vi "Report.vi"() -> ()   [LabVIEW 2017]
uses:
  <vilib>/Utility/miscctls.llb/LVRowAndColumnUnsignedTypeDef.ctl
  <vilib>/addons/database/Connection.llb/DB Tools Open Connec (String).vi
  <vilib>/Utility/file.llb/Write Delimited Spreadsheet (string).vi
  Global/Global 1.vi
  <vilib>/addons/database/NI_Database_API.lvlib
  <vilib>/Utility/NIReport.llb/NI_report.lvclass
  <vilib>/Utility/NIReport.llb/Append Text Table to Report (wrap).vi
panel:
  out "reposr save header":string[](array[string])
  in  "SELECT REPORT TYPE":string(combo)="WITHOUT TRECIABILITY"
  out "error out":errorcluster
  in  "error in (no error)":errorcluster
  in  "GET REPORT":bool
  in  "EXIT":bool
  in  "EXPORT TO EXCEL":bool
  in  "TO":timestamp format="%<%x>T"
  in  "FROM":timestamp format="%<%x>T"
  in  "BARCODE":string
  in  "TYPE":string(combo)="DATE TIME"
  in  "STATION WISE":string(combo)="OP 10"
  out "Table":string[][](table)
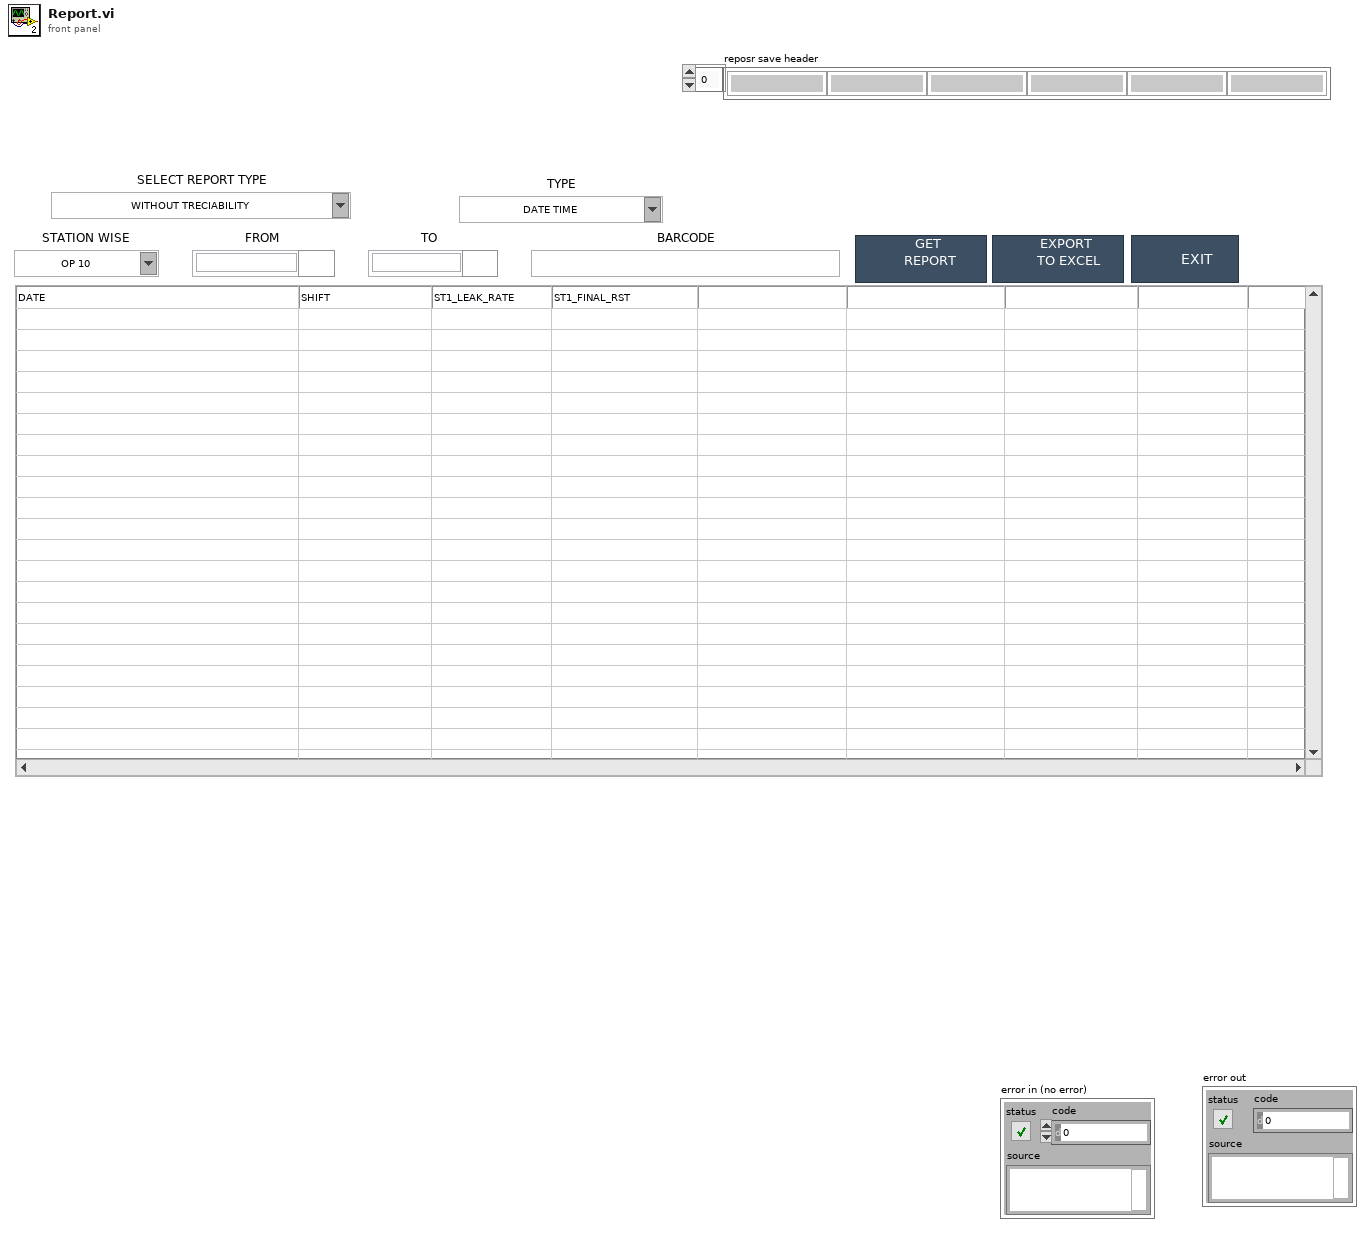
[diagram p1: front panel]
types:
  T1 = typedef "NI_Database_API.lvlib/Conn ObjectReference.ctl" = refnum<k1>
  T2 = typedef "LVRowAndColumnUnsignedTypeDef.ctl" = cluster{"Row":u32, "Column":u32}
  T3 = enum16{"Standard Report", "HTML", "Word", "Excel"}
  T4 = enum16{"maximized", "minimized", "normal", "no change"}
  T5 = enum32{"invalid app kind", "Development System", "Run Time System", "Student Edition", "Embedded LabVIEW", "Evaluation", "Custom"}
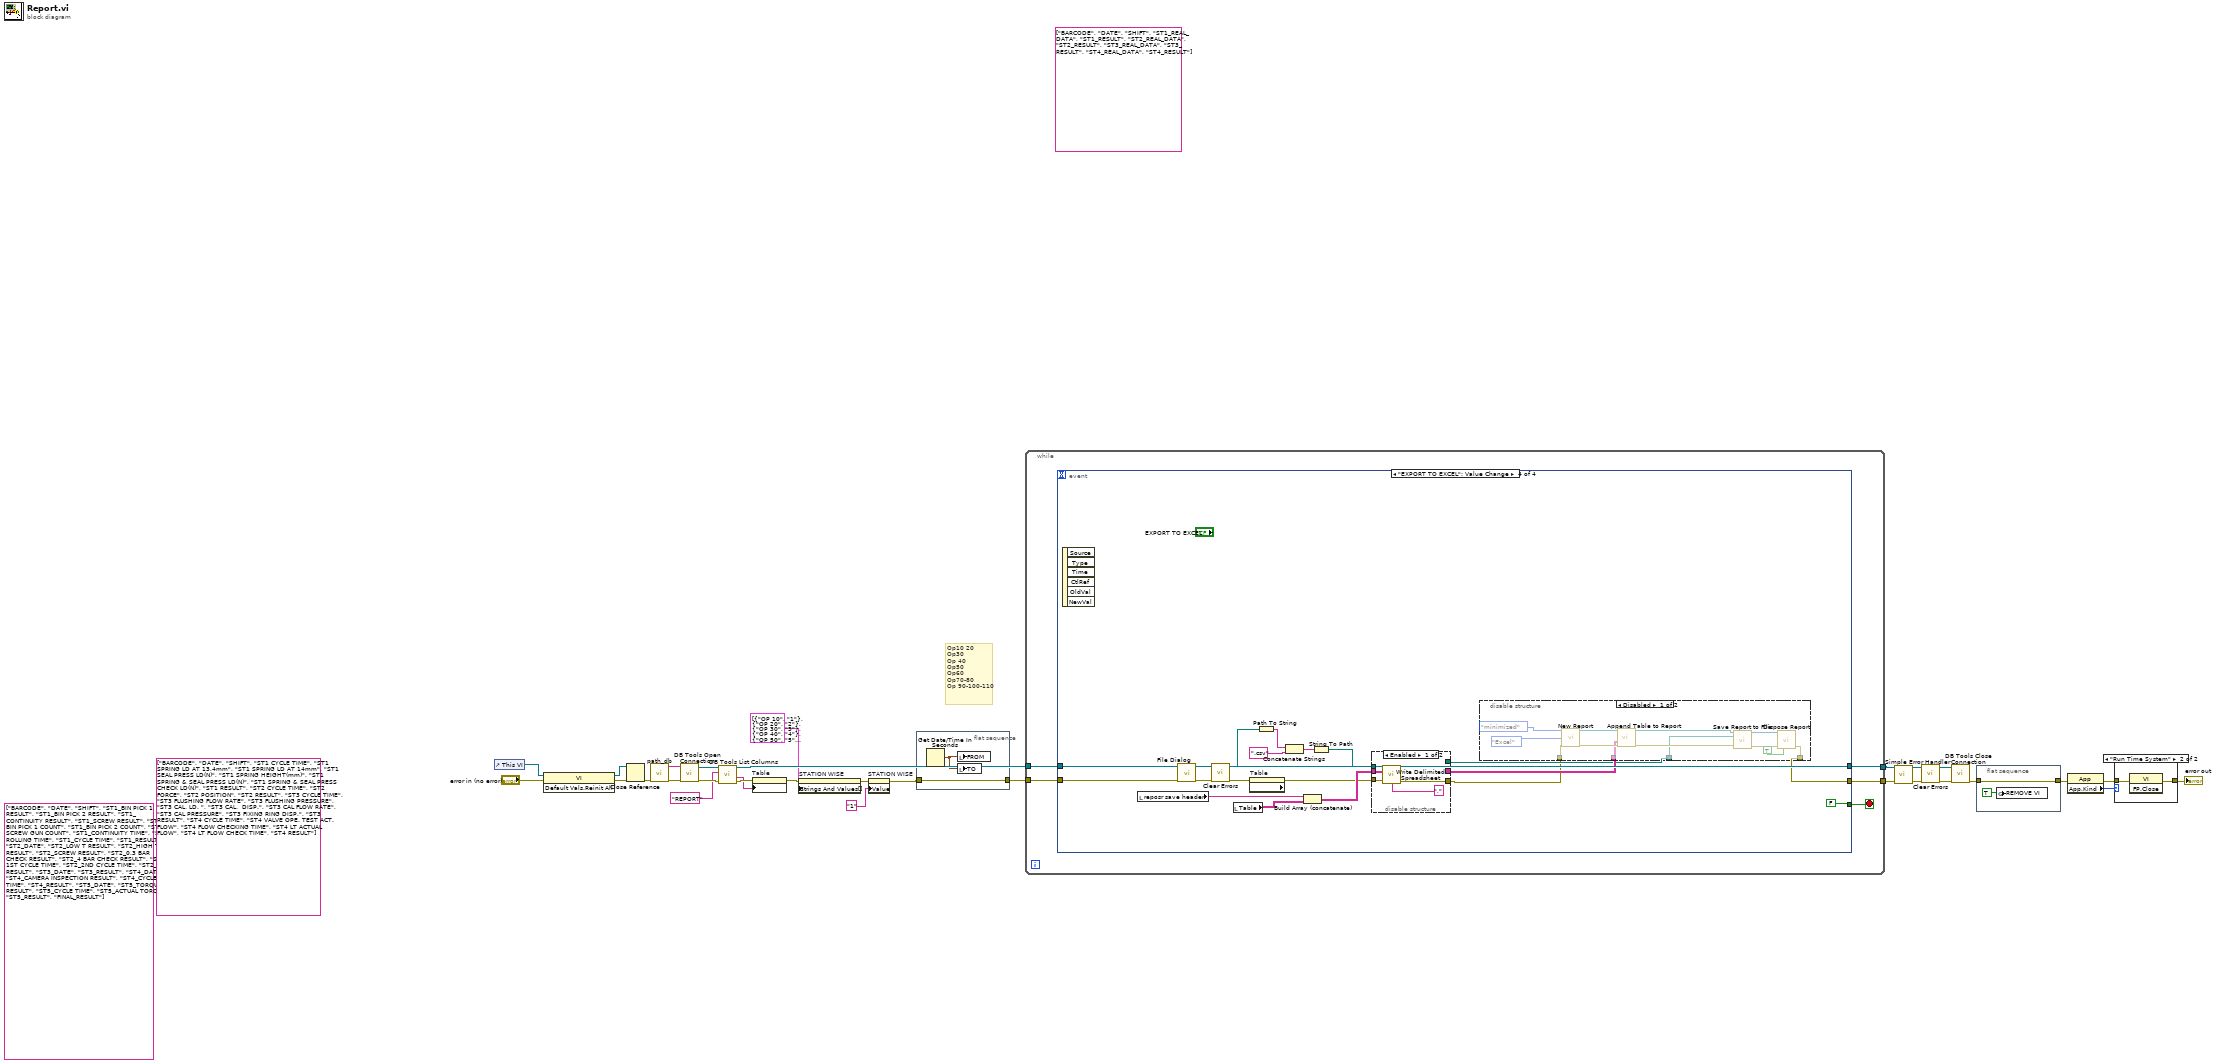
[diagram p0: block diagram]
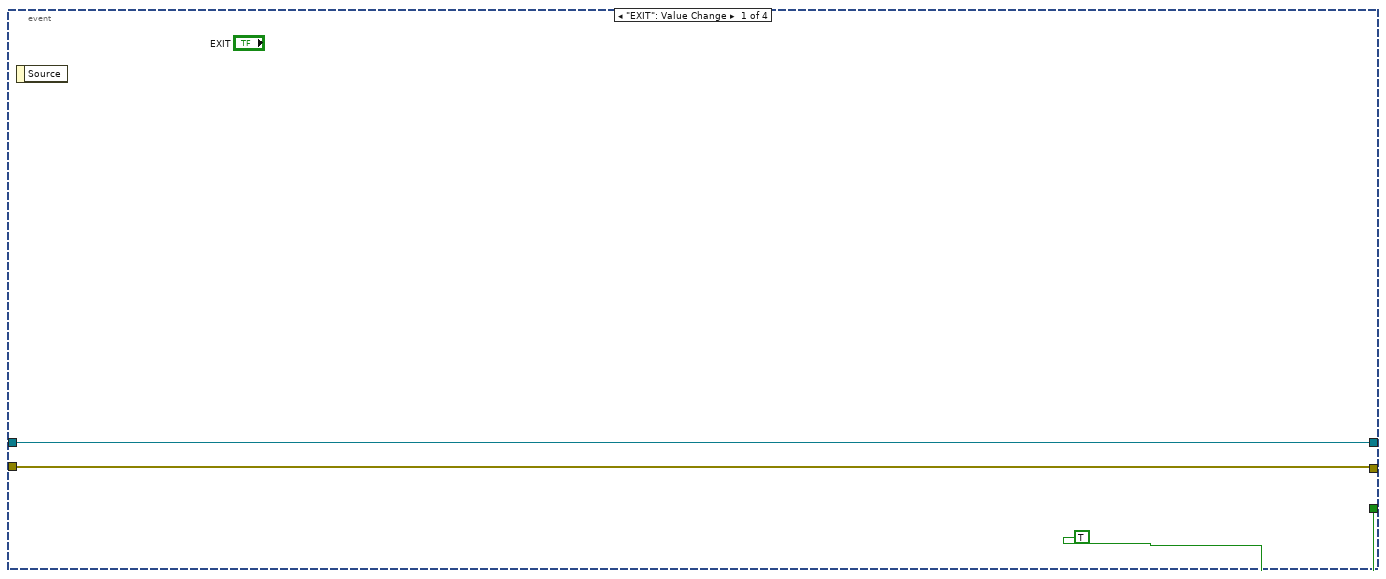
[diagram p2: hidden frame]
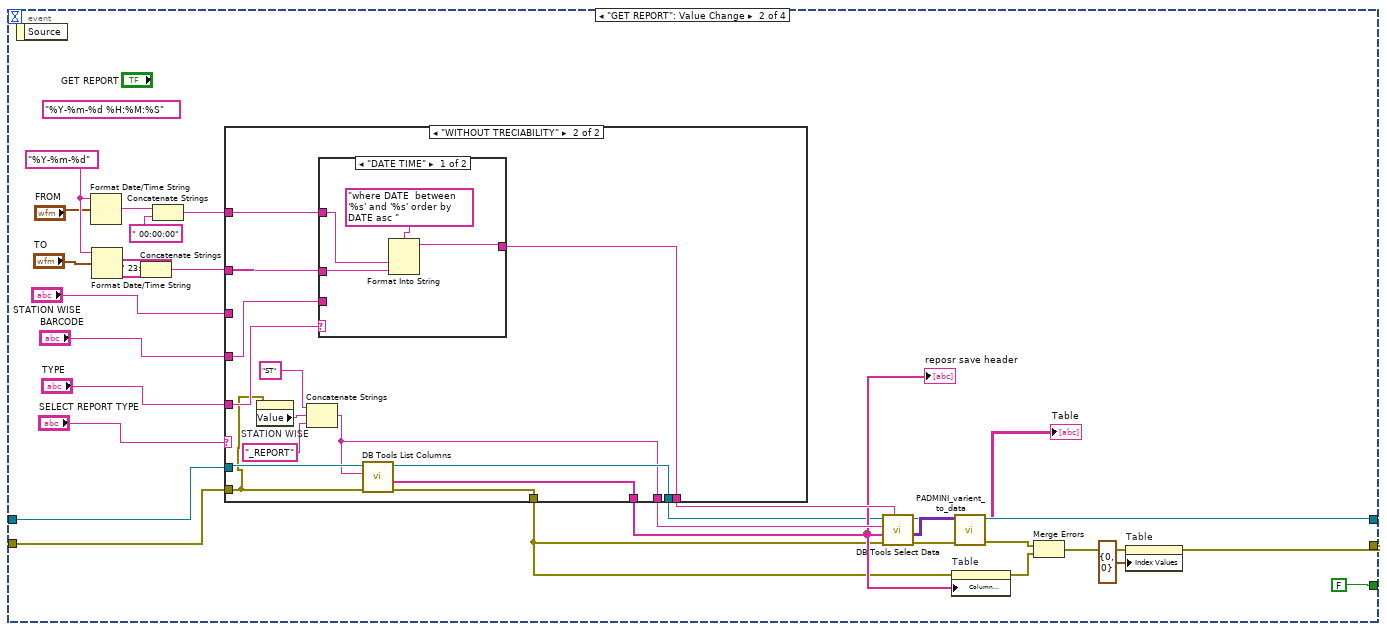
[diagram p3: hidden frame]
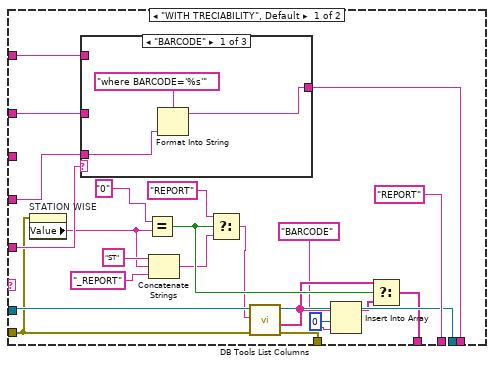
[diagram p4: hidden frame]
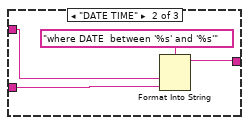
[diagram p5: hidden frame]
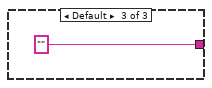
[diagram p6: hidden frame]
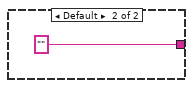
[diagram p7: hidden frame]
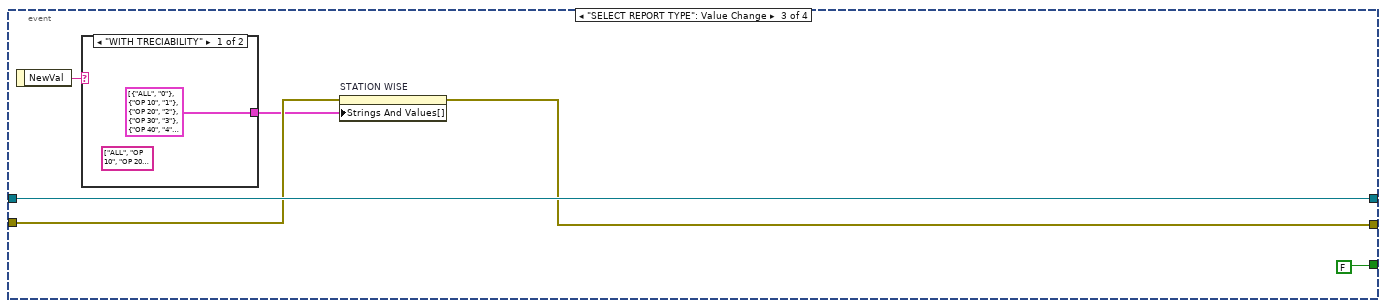
[diagram p8: hidden frame]
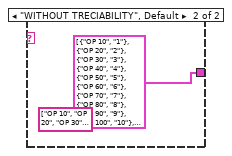
[diagram p9: hidden frame]
diagram:
  (unwired) string[] ["BARCODE", "DATE", "SHIFT", "ST1_REAL_DATA", "ST1_RESULT", "ST2_REAL_DATA", "ST2_RESULT", "ST3_REAL_DATA", "ST3_RESULT", "ST4_REAL_DATA", "ST4_RESULT"]
  (unwired) string[] ["BARCODE", "DATE", "SHIFT", "ST1_BIN PICK 1 RESULT", "ST1_BIN PICK 2 RESULT", "ST1_CONTINUITY RESULT", "ST1_SCREW RESULT", "ST1_BIN PICK 1 COUNT", "ST1_BIN PICK 2 COUNT", "ST1_SCREW GUN COUNT", "ST1_CONTINUITY TIME", "ST1_ROLLING TIME", "ST1_CYCLE TIME", "ST1_RESULT", "ST2_DATE", "ST2_LOW T RESULT", "ST2_HIGH T RESULT", "ST2_SCREW RESULT", "ST2_0.3 BAR CHECK RESULT", "ST2_4 BAR CHECK RESULT", "ST2_1ST CYCLE TIME", "ST2_2ND CYCLE TIME", "ST2_RESULT", "ST3_DATE", "ST3_RESULT", "ST4_DATE", "ST4_CAMERA INSPECTION RESULT", "ST4_CYCLE TIME", "ST4_RESULT", "ST5_DATE", "ST5_TORQUE RESULT", "ST5_CYCLE TIME", "ST5_ACTUAL TORQUE", "ST5_RESULT", "FINAL_RESULT"]
  (unwired) string[] ["BARCODE", "DATE", "SHIFT", "ST1 CYCLE TIME", "ST1 SPRING LD AT 13.4mm", "ST1 SPRING LD AT 14mm", "ST1 SEAL PRESS LD(N)", "ST1 SPRING HEIGHT(mm)", "ST1 SPRING & SEAL PRESS LD(N)", "ST1 SPRING & SEAL PRESS CHECK LD(N)", "ST1 RESULT", "ST2 CYCLE TIME", "ST2 FORCE", "ST2 POSITION", "ST2 RESULT", "ST3 CYCLE TIME", "ST3 FLUSHING FLOW RATE", "ST3 FLUSHING PRESSURE", "ST3 CAL. LD. ", "ST3 CAL.  DISP.", "ST3 CAL FLOW RATE", "ST3 CAL PRESSURE", "ST3 FIXING RING DISP.", "ST3 RESULT", "ST4 CYCLE TIME", "ST4 VALVE OPE. TEST ACT. FLOW", "ST4 FLOW CHECKING TIME", "ST4 LT ACTUAL FLOW", "ST4 LT FLOW CHECK TIME", "ST4 RESULT"]
  # "Op10 20\nOp30\nOp 40\nOp50\nOp60\nOp70-80\nOp 90-100-110"
  n1 = control-ref of="This VI"() -> (w28:refnum<vi>)
  n2 = invoke class="VI" method="Default Vals.Reinit All"(reference=w28, error in="error in (no error)") -> (reference out=w26:refnum<vi>, error out=w25:errorcluster)  [unwired: 1 in, 1 out]
  n3 = Close Reference(reference=w26, error in (no error)=w25) -> (error out=w15:errorcluster)
  n4 = call "path_db.vi"("error in"=w15) -> ("error out"=w17:errorcluster, "resulting string"=w16:string)  [unwired: 9 in]
  n5 = call-poly <vilib>:"DB Tools Open Connection.vi"("error in (no error)"=w17, "connection information"=w16) -> ("error out"=w10:errorcluster, "connection reference"=w7:T1)  [unwired: 6 in]
  n6 = call <vilib>:"DB Tools List Columns.vi"("error in (no error)"=w10, "table"="REPORT", "connection reference"=w7) -> ("error out"=w9:errorcluster, "columns"=w6:string[], "connection reference out"=w8:T1)  [unwired: 1 in, 1 out]
  n7 = property on="Table" class="Tbl (strict)"(error in=w9, "Column Headers[]"=w6) -> (error out=w12:errorcluster)  [unwired: 1 in, 1 out]
  n8 = property on="STATION WISE" class="CmbBox"(error in=w12, "Strings And Values[]"=cluster{"String":string, "Value":string}[] [{"String"="OP 10", "Value"="1"}, {"String"="OP 20", "Value"="2"}, {"String"="OP 30", "Value"="3"}, {"String"="OP 40", "Value"="4"}, {"String"="OP 50", "Value"="5"}, {"String"="OP 60", "Value"="6"}, {"String"="OP 70", "Value"="7"}, {"String"="OP 80", "Value"="8"}, {"String"="OP 90", "Value"="9"}, {"String"="OP 100", "Value"="10"}, {"String"="OP 110", "Value"="11"}] ("Strings And Values [] 2")) -> (error out=w3:errorcluster)  [unwired: 1 in, 1 out]
  n9 = property on="STATION WISE" class="CmbBox"(error in=w3, "Value"="1") -> (error out=w2:errorcluster)  [unwired: 1 in, 1 out]
  n10 = flat-sequence {
    tunnel: w2 -> [w29]
    tunnel: [w29] -> w11
    frame #0 {
      n11 = Get Date/Time In Seconds() -> (seconds since 1Jan1904=w30:timestamp)
      n12 = local write "FROM"(w30) -> ()
      n13 = local write "TO"(w30) -> ()
    }
  }
  n14 = while {
    tunnel: [w32] -> w18
    tunnel: w11 -> [w34]
    tunnel: w8 -> [w33]
    tunnel: [w31] -> w13
    stop <- w35 stop-if-true
    n15 = event shown="[3] \"EXPORT TO EXCEL\": Value Change" {
      selector: _ -> [_ _ _ _]
      dyn-events: _ -> [_ _ _ _]
      timeout: _ -> [_ _ _ _]
      tunnel: [TRUE FALSE FALSE FALSE] -> w35
      tunnel: w34 -> [w36 w45 w122 w132]
      tunnel: w33 -> [w37 w43 w124 w143]
      tunnel: [w37 w51 w124 w143] -> w31
      tunnel: [w36 w52 w119 w129] -> w32
      event "EXIT": Value Change {
        n16 = event-data() -> ()  [unwired: 1 in, 1 out]
      }
      event "GET REPORT": Value Change {
        (unwired) "%Y-%m-%d %H:%M:%S" ("time format string (%c)")
        w65 = "%Y-%m-%d" ("time format string (%c)")
        n17 = event-data() -> ()  [unwired: 1 in, 1 out]
        n18 = Format Date/Time String(time format string (%c)=w65, seconds (now)="FROM") -> (date/time string=w59:string)  [unwired: 1 in]
        n19 = Format Date/Time String(time format string (%c)=w65, seconds (now)="TO") -> (date/time string=w56:string)  [unwired: 1 in]
        n20 = Concatenate Strings(w56, " 23:59:59" ("time format string (%c)")) -> (w55:string)
        n21 = Concatenate Strings(w59, " 00:00:00" ("time format string (%c)")) -> (w58:string)
        n22 = case shown="\"WITHOUT TRECIABILITY\"" "SELECT REPORT TYPE" {
          tunnel: "TYPE" -> [w91 w113]
          tunnel: [w90 w112] -> w67
          tunnel: "BARCODE" -> [w89 w111]
          tunnel: w58 -> [w88 w110]
          tunnel: w55 -> [w87 w106]
          tunnel: "STATION WISE" -> [_ _]
          tunnel: ["REPORT" w101] -> w46
          tunnel: w45 -> [w69 w100]
          tunnel: [w83 w105] -> w39
          tunnel: [w79 w104] -> w44
          tunnel: w43 -> [w85 w103]
          tunnel: [w84 w102] -> w42
          frame "WITH TRECIABILITY", Default {
            n23 = property on="STATION WISE" class="CmbBox"(error in=w69) -> ("Value"=w70:string)  [unwired: 1 in, 2 out]
            n24 = case shown="\"BARCODE\"" w91 {
              tunnel: [w93 w97 ""] -> w90
              tunnel: w89 -> [w92 _ _]
              tunnel: w88 -> [_ w96 _]
              tunnel: w87 -> [_ w95 _]
              frame "BARCODE" {
                n25 = Format Into String(format string="where BARCODE='%s'", w92) -> (resulting string=w93:string)  [unwired: 2 in, 1 out]
              }
              frame "DATE TIME" {
                n26 = Format Into String(format string="where DATE  between '%s' and '%s'", w96, w95) -> (resulting string=w97:string)  [unwired: 2 in, 1 out]
              }
              frame Default {
              }
            }
            n27 = Equal?(x="0", y=w70) -> (x = y?=w81:bool)
            n28 = Concatenate Strings("ST", w70, "_REPORT") -> (w73:string)
            n29 = Select(t="REPORT", s=w81, f=w73) -> (s? t:f=w80:string)
            n30 = call <vilib>:"DB Tools List Columns.vi"("error in (no error)"=w69, "table"=w80, "connection reference"=w85) -> ("error out"=w83:errorcluster, "columns"=w78:string[], "connection reference out"=w84:T1)  [unwired: 1 in, 1 out]
            n31 = Insert Into Array(array=w78, index=0, new element="BARCODE" ("String")) -> (w76:string[])
            n32 = Select(t=w78, s=w81, f=w76) -> (s? t:f=w79:string[])
          }
          frame "WITHOUT TRECIABILITY" {
            n33 = property on="STATION WISE" class="CmbBox"(error in=w100) -> ("Value"=w109:string)  [unwired: 1 in, 2 out]
            n34 = Concatenate Strings("ST", w109, "_REPORT") -> (w101:string)
            n35 = case shown="\"DATE TIME\"" w113 {
              tunnel: [w117 ""] -> w112
              tunnel: w111 -> [_ _]
              tunnel: w110 -> [w116 _]
              tunnel: w106 -> [w115 _]
              frame "DATE TIME" {
                n36 = Format Into String(format string="where DATE  between '%s' and '%s' order by DATE asc ", w116, w115) -> (resulting string=w117:string)  [unwired: 2 in, 1 out]
              }
              frame Default {
              }
            }
            n37 = call <vilib>:"DB Tools List Columns.vi"("error in (no error)"=w100, "table"=w101, "connection reference"=w103) -> ("error out"=w105:errorcluster, "columns"=w104:string[], "connection reference out"=w102:T1)  [unwired: 1 in, 1 out]
          }
        }
        "reposr save header" <- w44
        n38 = call <vilib>:"DB Tools Select Data.vi"("condition"=w67, "error in (no error)"=w39, "columns"=w44, "table"=w46, "connection reference"=w42) -> ("error out"=w49:errorcluster, "data"=w54:variant[][], "connection reference out"=w51:T1)  [unwired: 1 in]
        n39 = property on="Table" class="Tbl (strict)"(error in=w39, "Column Headers[]"=w44) -> (error out=w48:errorcluster)  [unwired: 1 in, 1 out]
        n40 = call "PADMINI_varient_to_data.vi"("error in (no error)"=w49, "data"=w54) -> ("error out"=w47:errorcluster, "Array"=→"Table":string[][])  [unwired: 8 in]
        n41 = Merge Errors(w47, w48) -> (w53:errorcluster)
        n42 = property on="Table" class="Tbl (strict)"(error in=w53, "Index Values"=T2 {"Row"=0, "Column"=0}) -> (error out=w52:errorcluster)  [unwired: 1 in, 1 out]
      }
      event "SELECT REPORT TYPE": Value Change {
        n43 = event-data() -> ("NewVal"=w123:string)  [unwired: 1 in]
        n44 = case shown="\"WITH TRECIABILITY\"" w123 {
          tunnel: [cluster{"String":string, "Value":string}[] [{"String"="ALL", "Value"="0"}, {"String"="OP 10", "Value"="1"}, {"String"="OP 20", "Value"="2"}, {"String"="OP 30", "Value"="3"}, {"String"="OP 40", "Value"="4"}, {"String"="OP 50", "Value"="5"}, {"String"="OP 60", "Value"="6"}, {"String"="OP 70", "Value"="7"}, {"String"="OP 80", "Value"="8"}, {"String"="OP 90", "Value"="9"}, {"String"="OP 100", "Value"="10"}, {"String"="OP 110", "Value"="11"}] ("Strings And Values [] 2") cluster{"String":string, "Value":string}[] [{"String"="OP 10", "Value"="1"}, {"String"="OP 20", "Value"="2"}, {"String"="OP 30", "Value"="3"}, {"String"="OP 40", "Value"="4"}, {"String"="OP 50", "Value"="5"}, {"String"="OP 60", "Value"="6"}, {"String"="OP 70", "Value"="7"}, {"String"="OP 80", "Value"="8"}, {"String"="OP 90", "Value"="9"}, {"String"="OP 100", "Value"="10"}, {"String"="OP 110", "Value"="11"}] ("Strings And Values [] 2")] -> w120
          frame "WITH TRECIABILITY" {
            (unwired) string[] ["ALL", "OP 10", "OP 20", "OP 30", "OP 40", "OP 50", "OP 60", "OP 70", "OP 80", "OP 90", "OP 100", "OP 110"] ("Strings []")
          }
          frame "WITHOUT TRECIABILITY", Default {
            (unwired) string[] ["OP 10", "OP 20", "OP 30", "OP 40", "OP 50", "OP 60", "OP 70", "OP 80", "OP 90", "OP 100", "OP 110"] ("Strings []")
          }
        }
        n45 = property on="STATION WISE" class="CmbBox"(error in=w122, "Strings And Values[]"=w120) -> (error out=w119:errorcluster)  [unwired: 1 in, 1 out]
      }
      event "EXPORT TO EXCEL": Value Change {
        n46 = event-data() -> ()  [unwired: 1 in, 6 out]
        n47 = local read "reposr save header"() -> (w127:string[])
        n48 = call "File Dialog"("error in"=w132) -> ("selected path"=w141:path, "error out"=w142:errorcluster)  [unwired: 11 in, 2 out]
        n49 = call <vilib>:"Clear Errors.vi"("error in (no error)"=w142) -> ("error out"=w135:errorcluster)  [unwired: 5 in, 1 out]
        n50 = local read "Table"() -> (w144:string[][])
        n51 = property on="Table" class="Tbl (strict)" props=["Column Headers[]"](error in=w135) -> (error out=w134:errorcluster)  [unwired: 1 in, 2 out]
        n52 = Path To String(path=w141) -> (string=w140:string)
        n53 = Concatenate Strings(w140, ".csv" ("string")) -> (w138:string)
        n54 = Build Array (concatenate)(w127, w144) -> (w136:string[][])
        n55 = String To Path(string=w138) -> (path=w137:path)
        n56 = disable-structure shown="Enabled" {
          disable-tunnel: w137 -> [w163 w164]
          disable-tunnel: [w162 w166] -> w128
          disable-tunnel: w136 -> [w161 w165]
          disable-tunnel: w134 -> [w159 w166]
          disable-tunnel: [_ w165] -> w131
          disable-tunnel: [_ w164] -> w130
          frame Enabled {
            n57 = call-poly <vilib>:"Write Delimited Spreadsheet.vi"("file path (dialog if empty)"=w163, "2D data"=w161, "error in (no error)"=w159, "delimiter (\\t)"="," ("delimiter (\\t)")) -> ("error out"=w162:errorcluster)  [unwired: 10 in, 1 out]
          }
          frame Disabled {
          }
        }
        n58 = disable-structure shown="Disabled" {
          disable-tunnel: w131 -> [w148 _]
          disable-tunnel: w130 -> [w147 _]
          disable-tunnel: [w146 w158] -> w129
          disable-tunnel: w128 -> [w145 w158]
          frame Disabled {
            n59 = call <vilib>:"New Report.vi"("window state (normal)"=T4."minimized", "report type"=T3."Excel", "error in (no error)"=w145) -> ("report out"=w155:refnum<class "NI_report.lvclass">, "error out"=w154:errorcluster)  [unwired: 11 in]
            n60 = call-poly <vilib>:"Append Table to Report.vi"("report in"=w155, "text data"=w148, "error in (no error)"=w154) -> ("report out"=w151:refnum<class "NI_report.lvclass">, "error out"=w153:errorcluster)  [unwired: 9 in, 2 out]
            n61 = call-dynamic "Save Report to File.vi"("report in"=w151, "report file path"=w147, "error in (no error)"=w153) -> ("report out"=w150:refnum<class "NI_report.lvclass">, "error out"=w152:errorcluster)  [unwired: 11 in]
            n62 = call-dynamic "Dispose Report.vi"("report in"=w150, "error in (no error)"=w152, "close report? (T)"=TRUE) -> ("error out"=w146:errorcluster)  [unwired: 12 in]
          }
          frame Enabled {
          }
        }
      }
    }
  }
  n63 = call <vilib>:"Simple Error Handler.vi"("error in (no error)"=w18) -> ("error out"=w24:errorcluster)  [unwired: 4 in, 4 out]
  n64 = call <vilib>:"Clear Errors.vi"("error in (no error)"=w24) -> ("error out"=w23:errorcluster)  [unwired: 5 in, 1 out]
  n65 = call <vilib>:"DB Tools Close Connection.vi"("error in (no error)"=w23, "connection reference"=w13) -> ("error out"=w14:errorcluster)  [unwired: 5 in]
  n66 = flat-sequence {
    tunnel: [w168] -> w22
    tunnel: w14 -> [w168]
    frame #0 {
      n67 = global write "Global 1.vi" "REMOVE VI"(TRUE ("REMOVE VI")) -> ()
    }
  }
  n68 = property class="App"(error in=w22) -> (error out=w21:errorcluster, "App.Kind"=w20:T5)  [unwired: 1 in, 1 out]
  n69 = case shown="\"Run Time System\"" w20 {
    tunnel: w21 -> [w169 w171]
    tunnel: [w169 w170] -> w19
    frame "Development System", Default {
    }
    frame "Run Time System" {
      n70 = invoke class="VI" method="FP.Close"(error in=w171) -> (error out=w170:errorcluster)  [unwired: 2 in, 2 out]
    }
  }
  "error out" <- w19
